vi "SensorManipulationSubVI.vi"(11 "Array in":dbl[](array[numeric])) -> (3 "Array out":i32[](array[numeric]))   [LabVIEW 2021]
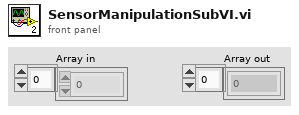
[diagram p1: front panel]
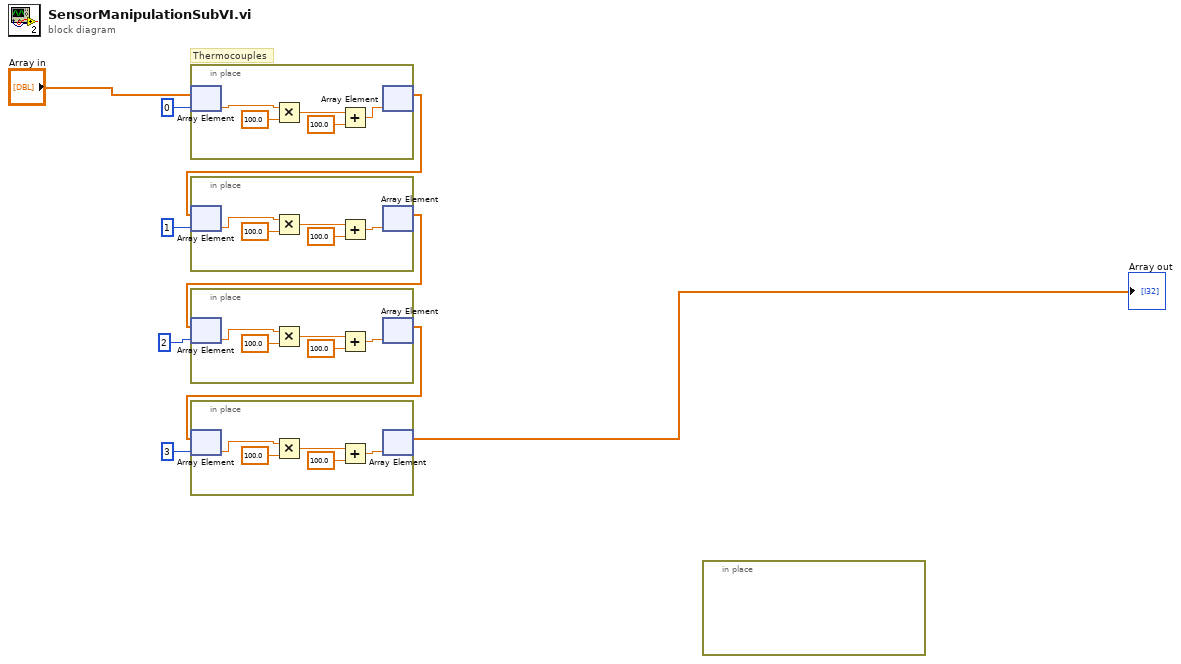
[diagram p0: block diagram]
diagram:
  # "Thermocouples"
  n1 = in-place {
    n2 = in-place-array #1("Array in", 0) -> (w11:dbl)
    n3 = Multiply(x=w11, y=100.0) -> (x*y=w14:dbl)
    n4 = Add(x=w14, y=100.0) -> (x+y=w10:dbl)
    n5 = in-place-array #1(w10) -> (w8:dbl[])  [unwired: 1 out]
  }
  n6 = in-place {
    n7 = in-place-array #2(w8, 1) -> (w16:dbl)
    n8 = Multiply(x=w16, y=100.0) -> (x*y=w19:dbl)
    n9 = Add(x=w19, y=100.0) -> (x+y=w15:dbl)
    n10 = in-place-array #2(w15) -> (w7:dbl[])  [unwired: 1 out]
  }
  n11 = in-place {
    n12 = in-place-array #3(w7, 2) -> (w21:dbl)
    n13 = Multiply(x=w21, y=100.0) -> (x*y=w24:dbl)
    n14 = Add(x=w24, y=100.0) -> (x+y=w20:dbl)
    n15 = in-place-array #3(w20) -> (w6:dbl[])  [unwired: 1 out]
  }
  n16 = in-place {
    n17 = in-place-array #4(w6, 3) -> (w26:dbl)
    n18 = Multiply(x=w26, y=100.0) -> (x*y=w29:dbl)
    n19 = Add(x=w29, y=100.0) -> (x+y=w25:dbl)
    n20 = in-place-array #4(w25) -> (→"Array out":dbl[])  [unwired: 1 out]
  }
  n21 = in-place {
  }
